vi "onAssertionSlippage.vi"(7 "AssertEqualValue in":refnum<class "AssertError.lvclass">, 10 "Properties":refnum<class "Properties.Assert.lvclass">) -> (0 "error out":errorcluster, 2 "Properties out":refnum<class "Properties.Assert.lvclass">)   [LabVIEW 2021, in "Bananas.lvlib" / "AssertError.lvclass"]
uses:
  AssertError.lvclass
  <vilib>/addons/_JKI Toolkits/Caraya/classes/Properties.Assert/Properties.Assert.lvclass
  C:/Program Files (x86)/National Instruments/LabVIEW 2021/vi.lib/addons/_JKI Toolkits/Caraya/classes/Properties/Properties.lvclass
  <vilib>/addons/_JKI Toolkits/Caraya/classes/Properties.Assert/Properties.Assert.lvclass/Properties.Assert.ctl
  AssertError.lvclass/AssertError.ctl
  <vilib>/Utility/error.llb/DialogType.ctl
  Read Not_.vi
  Read Error.vi
  <vilib>/addons/_JKI Toolkits/Caraya/classes/Properties/Properties.lvclass
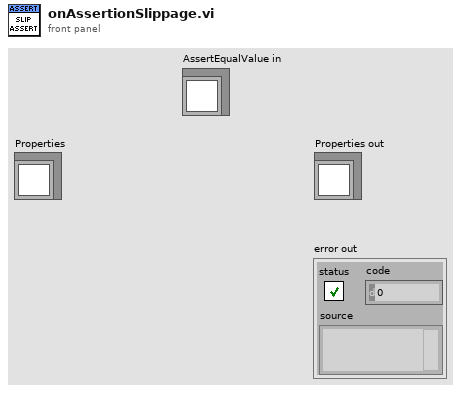
[diagram p1: front panel]
types:
  T1 = typedef "DialogType.ctl" = u16
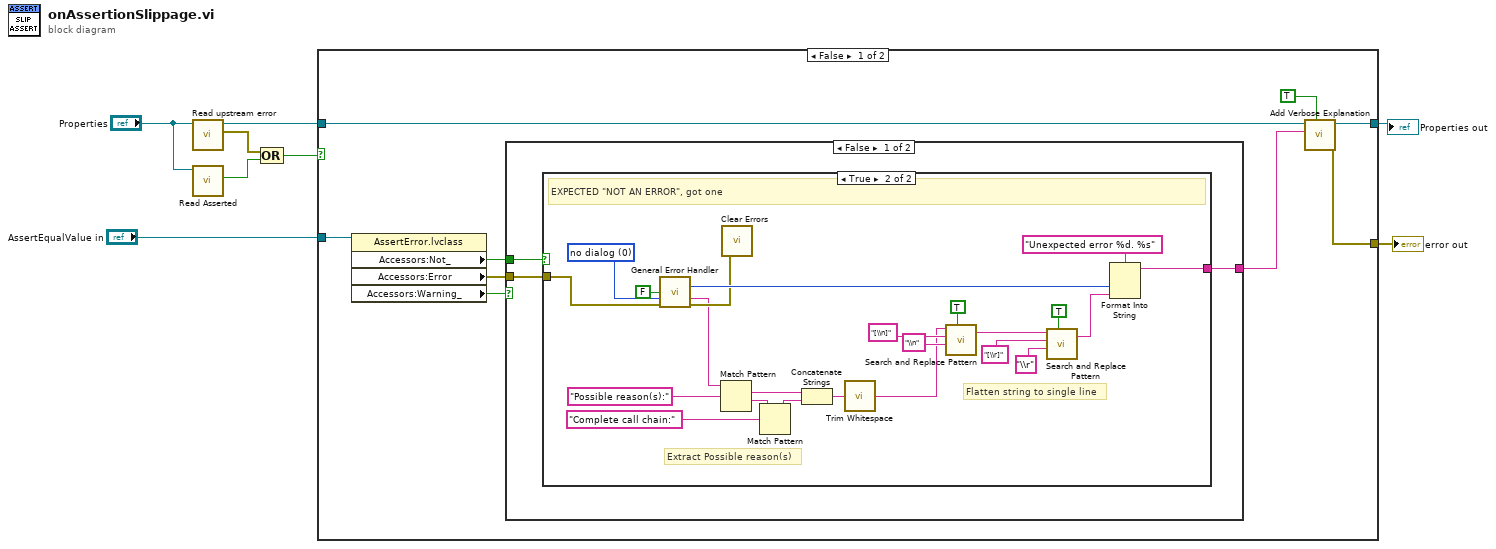
[diagram p0: block diagram]
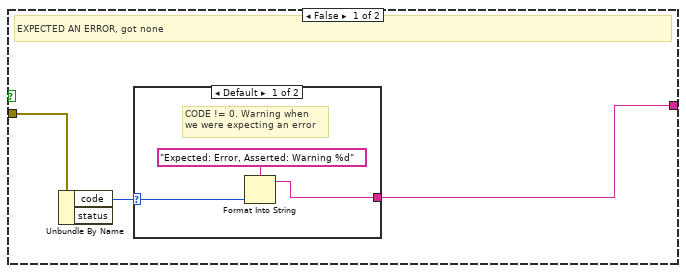
[diagram p2: hidden frame]
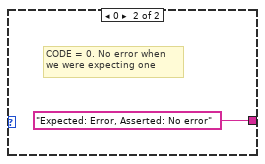
[diagram p3: hidden frame]
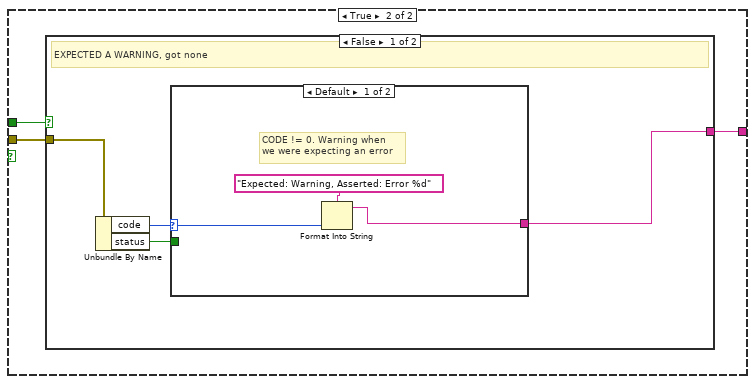
[diagram p4: hidden frame]
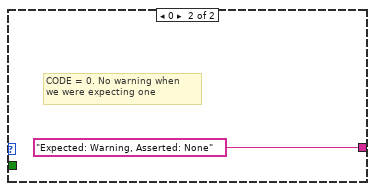
[diagram p5: hidden frame]
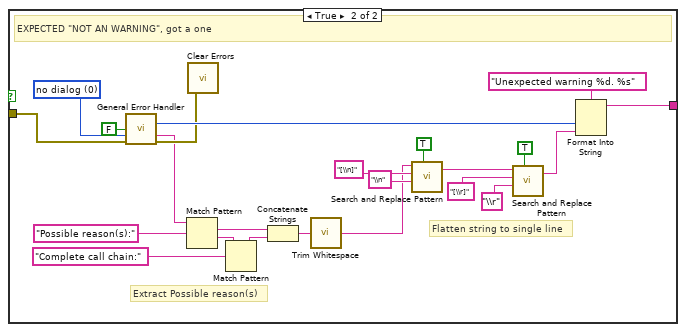
[diagram p6: hidden frame]
diagram:
  n1 = call <vilib>:"Read upstream error.vi"("Properties.Assert in"="Properties") -> ("upstream-error"=w7:errorcluster, "Properties.Assert out"=w8:refnum<class "Properties.Assert.lvclass">)  [unwired: 9 in]
  n2 = call <vilib>:"Read Asserted.vi"("Properties.Assert in"="Properties") -> ("Asserted"=w6:bool)  [unwired: 9 in, 1 out]
  n3 = Compound Arithmetic op=OR(w7, w6) -> (w5:bool)
  n4 = case shown="False" w5 {
    tunnel: [w16 w85] -> w3
    tunnel: [w15 _] -> w2
    tunnel: w8 -> [w17 w85]
    tunnel: "AssertEqualValue in" -> [w13 _]
    frame False {
      n5 = property class="AssertError.lvclass"(reference=w13) -> ("Accessors:Not_"=w11:bool, "Accessors:Error"=w10:errorcluster, "Accessors:Warning_"=w9:bool)  [unwired: 1 in, 2 out]
      n6 = case shown="False" w9 {
        tunnel: [w20 w53] -> w12
        tunnel: w11 -> [w19 w52]
        tunnel: w10 -> [w18 w51]
        frame False {
          n7 = case shown="True" w19 {
            tunnel: [w21 w50] -> w20
            tunnel: w18 -> [w23 w48]
            frame False {
              # "EXPECTED AN ERROR, got none"
              n8 = Unbundle By Name(w23) -> ("code"=w22:i32)  [unwired: 1 out]
              n9 = case shown="Default" w22 {
                selector: w22 -> [w26 _]
                tunnel: [w24 "Expected: Error, Asserted: No error"] -> w21
                frame Default {
                  # "CODE != 0. Warning when \nwe were expecting an error"
                  n10 = Format Into String(format string="Expected: Error, Asserted: Warning %d", w26) -> (resulting string=w24:string)  [unwired: 2 in, 1 out]
                }
                frame 0 {
                  # "CODE = 0. No error when \nwe were expecting one"
                }
              }
            }
            frame True {
              w47 = T1 0 items=["no dialog", "OK message", "continue or stop message", "OK message + warnings", "continue/stop + warnings"] ("type of dialog (OK msg:1)")
              # "Extract Possible reason(s)"
              # "Flatten string to single line"
              # "EXPECTED \"NOT AN ERROR\", got one"
              n11 = call <vilib>:"General Error Handler.vi"("search ni.com link visible?(T)"=FALSE, "type of dialog (OK msg:1)"=w47, "error in (no error)"=w48) -> ("code out"=w46:i32, "message"=w39:string, "error out"=w45:errorcluster)  [unwired: 8 in, 2 out]
              n12 = Match Pattern(string=w39, regular expression="Possible reason(s):") -> (match substring=w31:string, after substring=w38:string)  [unwired: 1 in, 2 out]
              n13 = call <vilib>:"Clear Errors.vi"("error in (no error)"=w45) -> ()  [unwired: 5 in, 2 out]
              n14 = Match Pattern(string=w38, regular expression="Complete call chain:") -> (before substring=w30:string)  [unwired: 1 in, 3 out]
              n15 = Concatenate Strings(w31, w30) -> (w29:string)
              n16 = call <vilib>:"Trim Whitespace.vi"("string"=w29) -> ("trimmed string"=w28:string)  [unwired: 1 in]
              n17 = call <vilib>:"Search and Replace Pattern.vi"("string"=w28, "regular expression (\"\")"="[\\n]", "replace string (\"\")"="\\n", "replace all? (F)"=TRUE) -> ("result string"=w35:string)  [unwired: 1 in, 1 out]
              n18 = call <vilib>:"Search and Replace Pattern.vi"("string"=w35, "regular expression (\"\")"="[\\r]", "replace string (\"\")"="\\r", "replace all? (F)"=TRUE) -> ("result string"=w34:string)  [unwired: 1 in, 1 out]
              n19 = Format Into String(format string="Unexpected error %d. %s", w46, w34) -> (resulting string=w50:string)  [unwired: 2 in, 1 out]
            }
          }
        }
        frame True {
          n20 = case shown="False" w52 {
            tunnel: [w55 w84] -> w53
            tunnel: w51 -> [w57 w82]
            frame False {
              # "EXPECTED A WARNING, got none"
              n21 = Unbundle By Name(w57) -> ("code"=w56:i32, "status"=w54:bool)
              n22 = case shown="Default" w56 {
                selector: w56 -> [w60 _]
                tunnel: [w58 "Expected: Warning, Asserted: None"] -> w55
                tunnel: w54 -> [_ _]
                frame Default {
                  # "CODE != 0. Warning when \nwe were expecting an error"
                  n23 = Format Into String(format string="Expected: Warning, Asserted: Error %d", w60) -> (resulting string=w58:string)  [unwired: 2 in, 1 out]
                }
                frame 0 {
                  # "CODE = 0. No warning when \nwe were expecting one"
                }
              }
            }
            frame True {
              w81 = T1 0 items=["no dialog", "OK message", "continue or stop message", "OK message + warnings", "continue/stop + warnings"] ("type of dialog (OK msg:1)")
              # "Extract Possible reason(s)"
              # "Flatten string to single line"
              # "EXPECTED \"NOT AN WARNING\", got a one"
              n24 = call <vilib>:"General Error Handler.vi"("search ni.com link visible?(T)"=FALSE, "type of dialog (OK msg:1)"=w81, "error in (no error)"=w82) -> ("code out"=w80:i32, "message"=w73:string, "error out"=w79:errorcluster)  [unwired: 8 in, 2 out]
              n25 = Match Pattern(string=w73, regular expression="Possible reason(s):") -> (match substring=w65:string, after substring=w72:string)  [unwired: 1 in, 2 out]
              n26 = call <vilib>:"Clear Errors.vi"("error in (no error)"=w79) -> ()  [unwired: 5 in, 2 out]
              n27 = Match Pattern(string=w72, regular expression="Complete call chain:") -> (before substring=w64:string)  [unwired: 1 in, 3 out]
              n28 = Concatenate Strings(w65, w64) -> (w63:string)
              n29 = call <vilib>:"Trim Whitespace.vi"("string"=w63) -> ("trimmed string"=w62:string)  [unwired: 1 in]
              n30 = call <vilib>:"Search and Replace Pattern.vi"("string"=w62, "regular expression (\"\")"="[\\n]", "replace string (\"\")"="\\n", "replace all? (F)"=TRUE) -> ("result string"=w69:string)  [unwired: 1 in, 1 out]
              n31 = call <vilib>:"Search and Replace Pattern.vi"("string"=w69, "regular expression (\"\")"="[\\r]", "replace string (\"\")"="\\r", "replace all? (F)"=TRUE) -> ("result string"=w68:string)  [unwired: 1 in, 1 out]
              n32 = Format Into String(format string="Unexpected warning %d. %s", w80, w68) -> (resulting string=w84:string)  [unwired: 2 in, 1 out]
            }
          }
        }
      }
      n33 = call <vilib>:"Add Verbose Explanation.vi"("overwrite?"=TRUE, "Verbose Explanation"=w12, "Properties"=w17) -> ("error out"=w15:errorcluster, "Properties"=w16:refnum<class "Properties.Assert.lvclass">)  [unwired: 7 in]
    }
    frame True {
      # "There was an upstream error or the assertion = TRUE"
    }
  }
  "error out" <- w2
  "Properties out" <- w3
